vi "TranslateTyping.vi"(11 "Cluster":T2) -> (1 "Script?":bool, 3 "string":string)   [LabVIEW 2016]
uses:
  <vilib>/event_ctls.llb/eventvkey.ctl
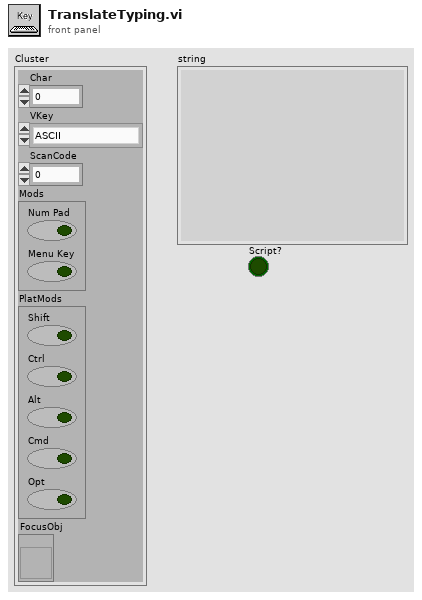
[diagram p1: front panel]
types:
  T1 = typedef "eventvkey.ctl" = enum16{"ASCII", "Enter", "Return", "Shift", "Ctrl", "Alt", "Cmd", "Opt", "Caps", "NumLock", "Clear", "Break", "Up", "Down", "Left", "Right", "Insert", "Delete", "Home", "End", "PageUp", "PageDown", "Escape", "Help", "Pause", "ScrollLock", "F1", "F2", "F3", "F4", "F5", "F6", "F7", "F8", "F9", "F10", "F11", "F12", "F13", "F14", "F15", "F16", "F17", "F18", "F19", "F20", "F21", "F22", "F23", "F24", "Play", "VolumeUp", "VolumeDown", "Mute", "Two Byte Char"}
  T2 = cluster{"Char":i16, "VKey":T1, "ScanCode":i16, "Mods":cluster{"Num Pad":bool, "Menu Key":bool}, "PlatMods":cluster{"Shift":bool, "Ctrl":bool, "Alt":bool, "Cmd":bool, "Opt":bool}, "FocusObj":refnum<vi>}
  T3 = cluster{"Shift":bool, "Ctrl":bool, "Alt":bool, "Cmd":bool, "Opt":bool}
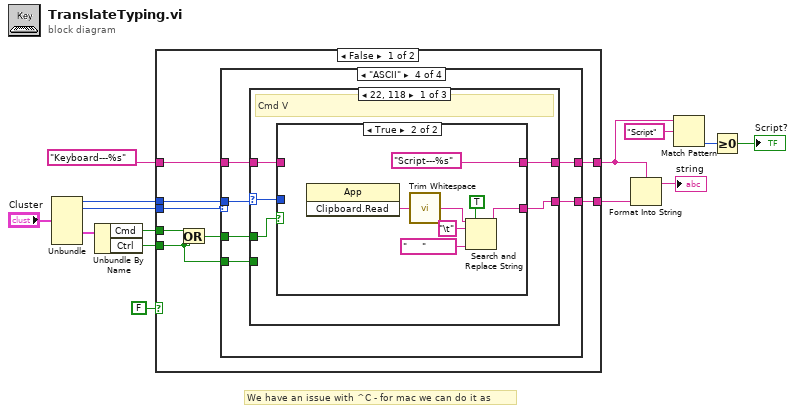
[diagram p0: block diagram]
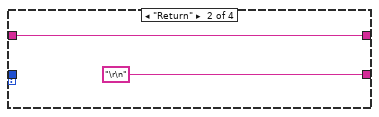
[diagram p3: hidden frame]
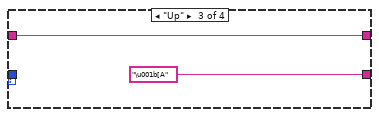
[diagram p4: hidden frame]
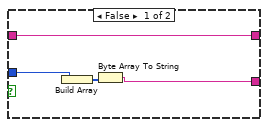
[diagram p5: hidden frame]
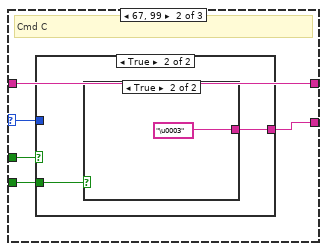
[diagram p6: hidden frame]
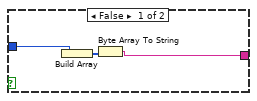
[diagram p7: hidden frame]
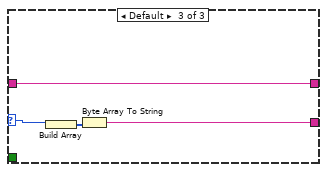
[diagram p9: hidden frame]
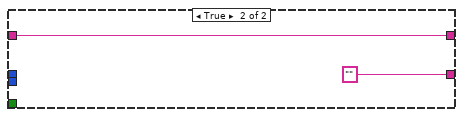
[diagram p10: hidden frame]
diagram:
  # "We have an issue with ^C - for mac we can do it as"
  n1 = Unbundle("Cluster") -> ("Char"=w13:i16, "VKey"=w12:T1, "PlatMods"=w11:T3)  [unwired: 3 out]
  n2 = Unbundle By Name(w11) -> ("Cmd"=w7:bool, "Ctrl"=w10:bool)
  n3 = case shown="False" FALSE {
    tunnel: [w22 "" ("string")] -> w9
    tunnel: w13 -> [w21 _]
    tunnel: w12 -> [w20 _]
    tunnel: w10 -> [w17 _]
    tunnel: w7 -> [w18 _]
    tunnel: [w16 w65] -> w4
    tunnel: "Keyboard---%s" -> [w15 w65]
    frame False {
      n4 = Or(x=w18, y=w17) -> (x .or. y?=w19:bool)
      n5 = case shown="\"ASCII\"" w20 {
        tunnel: [_ "\r\n" ("string") "\u001b[A" ("string") w33] -> w22
        tunnel: w21 -> [_ _ _ w32]
        tunnel: w19 -> [_ _ _ w31]
        tunnel: w17 -> [_ _ _ w30]
        tunnel: [w23 w24 w26 w29] -> w16
        tunnel: w15 -> [w23 w24 w26 w28]
        frame Default {
        }
        frame "Return" {
        }
        frame "Up" {
        }
        frame "ASCII" {
          n6 = case shown="22, 118" w32 {
            selector: w32 -> [w36 w52 w62]
            tunnel: [w38 w54 w64] -> w33
            tunnel: w31 -> [w37 w53 _]
            tunnel: w30 -> [_ w51 _]
            tunnel: [w35 w50 w61] -> w29
            tunnel: w28 -> [w34 w50 w61]
            frame 22, 118 {
              # "Cmd V"
              n7 = case shown="True" w37 {
                tunnel: [w40 w44] -> w38
                tunnel: w36 -> [w41 _]
                tunnel: [w39 "Script---%s"] -> w35
                tunnel: w34 -> [w39 _]
                frame False {
                  n8 = Build Array(w41) -> (w42:i16[])
                  n9 = Byte Array To String(unsigned byte array=w42) -> (string=w40:string)
                }
                frame True {
                  n10 = invoke class="App" method="Clipboard.Read"() -> ("Read Clipbrd"=w49:string)  [unwired: 3 in, 2 out]
                  n11 = call <vilib>:"Trim Whitespace.vi"("string"=w49) -> ("trimmed string"=w48:string)  [unwired: 1 in]
                  n12 = Search and Replace String(replace all?=TRUE ("replace all? (F)"), input string=w48, search string="\t", replace string="     " ("replace string (\"\")")) -> (result string=w44:string)  [unwired: 4 in, 3 out]
                }
              }
            }
            frame 67, 99 {
              # "Cmd C"
              n13 = case shown="True" w53 {
                tunnel: [w55 w58] -> w54
                tunnel: w52 -> [w56 _]
                tunnel: w51 -> [_ w59]
                frame False {
                  n14 = Build Array(w56) -> (w57:i16[])
                  n15 = Byte Array To String(unsigned byte array=w57) -> (string=w55:string)
                }
                frame True {
                  n16 = case shown="True" w59 {
                    tunnel: [_ "\u0003"] -> w58
                    frame False {
                    }
                    frame True {
                    }
                  }
                }
              }
            }
            frame Default {
              n17 = Build Array(w62) -> (w63:i16[])
              n18 = Byte Array To String(unsigned byte array=w63) -> (string=w64:string)
            }
          }
        }
      }
    }
    frame True {
    }
  }
  n19 = Format Into String(format string=w4, w9) -> (resulting string=→"string":string)  [unwired: 2 in, 1 out]
  n20 = Match Pattern(string=w4, regular expression="Script") -> (offset past match=w2:i32)  [unwired: 1 in, 3 out]
  n21 = Greater Or Equal To 0?(x=w2) -> (x >= 0?=→"Script?":bool)
